vi "DisableEnableStart.vi"() -> (0 "S2AckVisable":bool, 1 "S1AckVisable":bool, 2 "Station2":T1(ring), 3 "Station1":T1(ring))   [LabVIEW 2018, in "GUI.lvclass"]
uses:
  GUI.lvclass
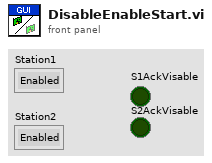
[diagram p1: front panel]
types:
  T1 = enum8{"Enabled", "Disabled", "Disabled and Grayed Out"}
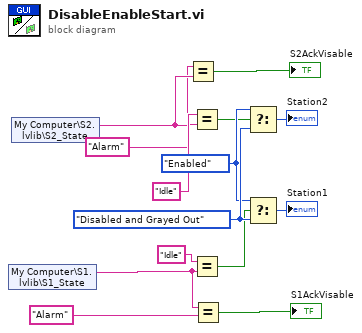
[diagram p0: block diagram]
diagram:
  w13 = T1."Disabled and Grayed Out" ("Disabled")
  w12 = T1."Enabled" ("Disabled")
  n1 = shared-variable "My Computer\\S1.lvlib\\S1_State"() -> (w5:string)  [unwired: 1 in, 1 out]
  n2 = shared-variable "My Computer\\S2.lvlib\\S2_State"() -> (w7:string)  [unwired: 1 in, 1 out]
  n3 = Equal?(x="Alarm" ("y"), y=w7) -> (x = y?=→"S2AckVisable":bool)
  n4 = Equal?(x="Idle" ("y"), y=w7) -> (x = y?=w11:bool)
  n5 = Equal?(x="Idle" ("y"), y=w5) -> (x = y?=w9:bool)
  n6 = Equal?(x=w5, y="Alarm") -> (x = y?=→"S1AckVisable":bool)
  n7 = Select(t=w12, s=w11, f=w13) -> (s? t:f=→"Station2":T1)
  n8 = Select(t=w12, s=w9, f=w13) -> (s? t:f=→"Station1":T1)
